vi "cluster_v08.vi"() -> ()   [LabVIEW 2009]
uses:
  <vilib>/Math Plots/2D Math Plots/2D Compass/2D Compass XCtrl/2D Compass.xctl
  <vilib>/Math Plots/2D Math Plots/2D Compass/2D Compass Datatype/Public/Plot Helper (Vector).vi
  <vilib>/Math Plots/2D Math Plots/2D Compass/2D Compass Datatype/2D Compass Datatype.lvclass
panel:
  out "2D Compass":refnum<class "2D Plot Datatype.lvclass">[](xcontrol)
  out "alfa":dbl
  in  "stop":bool
  in  "Slide":u8(slide) scale=0.0..5.0
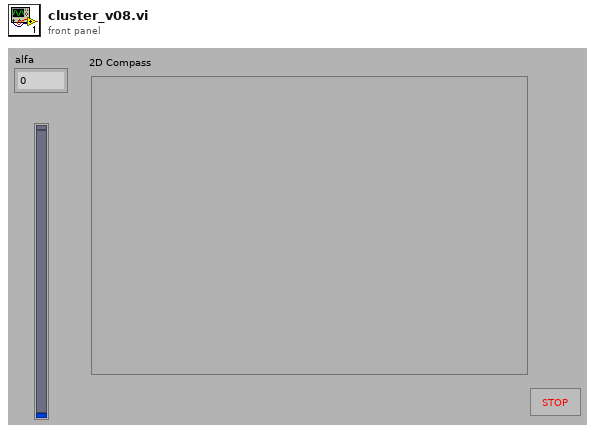
[diagram p1: front panel]
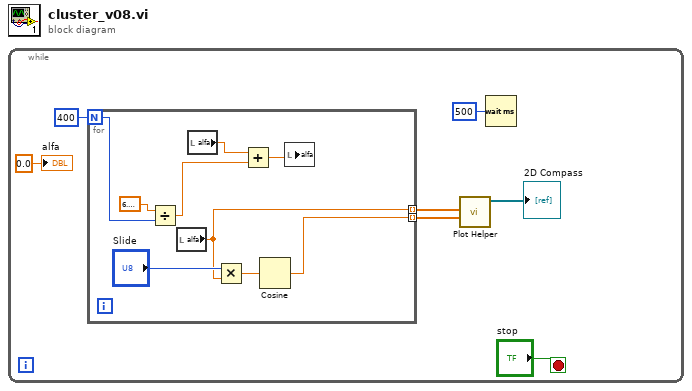
[diagram p0: block diagram]
diagram:
  n1 = while {
    stop <- "stop" stop-if-true
    n2 = for {
      N: 400 -> [w13]
      tunnel: [w8] -> w3 mode=indexing
      tunnel: [w14] -> w2 mode=indexing
      n3 = Divide(x=6.283185307179586, y=w13) -> (x/y=w9:dbl)
      n4 = local read "alfa"() -> (w8:dbl)
      n5 = local read "alfa"() -> (w10:dbl)
      n6 = Multiply(x="Slide", y=w8) -> (x*y=w16:dbl)
      n7 = Add(x=w10, y=w9) -> (x+y=w11:dbl)
      n8 = Cosine(x=w16) -> (cos(x)=w14:dbl)
      n9 = local write "alfa"(w11) -> ()
    }
    n10 = call-poly <vilib>:"Plot Helper.vi"("radius vector"=w2, "theta vector"=w3) -> ("2D Plot Class Obj Array out"=→"2D Compass":refnum<class "2D Plot Datatype.lvclass">[])  [unwired: 2 in, 7 out]
    n11 = Wait (ms)(milliseconds to wait=u32 500) -> ()  [unwired: 1 out]
    "alfa" <- 0.0 ("alfa")
  }
